vi "Load Process.vi"(0 "Object name":string, 3 "timeout (ms)":i32=10000, 5 "error in (no error)":errorcluster) -> (19 "error out":errorcluster)   [LabVIEW 2014, in "PTUtils.lvlib"]
uses:
  PTUtils.lvlib
  CS_Core/CSSystem/CoreDefs/CoreDefs.call_type.ctl
  CS_Core/BaseProcess/BaseProcess.descriptor string definition.ctl
  CS_Core/CSSystem/CoreDefs/CoreDefs.rawDataType.ctl
  CS_Core/CSSystem/CoreLib/CoreLib.string 2 byte array.vi
  CS_Core/CSSystem/CoreLib/CoreLib.lvlib
  CS_Core/CSSystem/CSSystemLib/CSSystemLib.lvlib
  CS_Core/BaseProcess/BaseProcess.lvlib
panel:
  in  "call cluster":T1
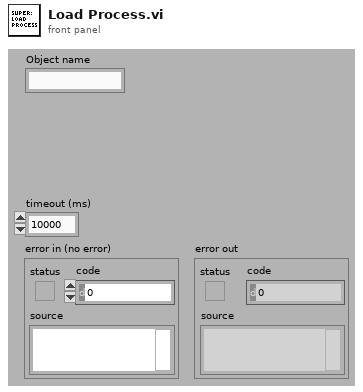
[diagram p1: front panel]
types:
  T1 = typedef "CoreDefs.call_type.ctl" = cluster{"Object":string, "Selector":string, "CallType":enum16{"simple", "synchronous", "asynchronous"}, "Async Object":string, "Async Selector":string, "Data Descriptor":T2, "Data":T3, "Error #":i32, "Expire":u32}
  T2 = typedef "BaseProcess.lvlib/BaseProcess.descriptor string definition.ctl" = string
  T3 = typedef "CoreDefs.rawDataType.ctl" = i8[]
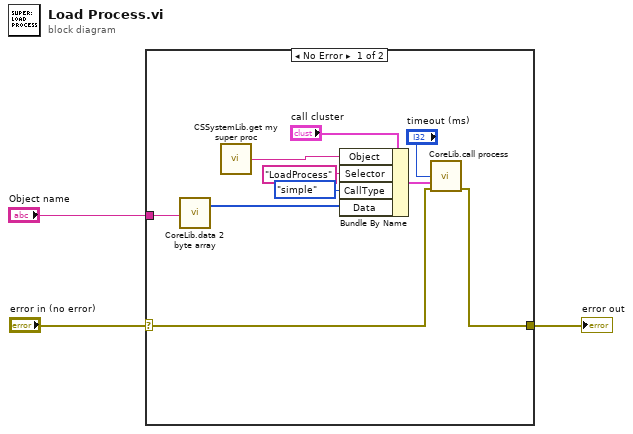
[diagram p0: block diagram]
diagram:
  n1 = case shown="No Error" "error in (no error)" {
    selector: "error in (no error)" -> [w6 w14]
    tunnel: "Object name" -> [w4 _]
    tunnel: [w5 w14] -> w1
    frame No Error {
      n2 = call-poly "CoreLib.data 2 byte array.vi"("string"=w4) -> ("byteArray out"=w13:T3)  [unwired: 18 in]
      n3 = call "CSSystemLib.get my super proc.vi"() -> ("name"=w10:string)  [unwired: 1 in]
      n4 = Bundle By Name(cluster="call cluster", "Object"=w10, "Selector"="LoadProcess", "CallType"=enum16{"simple", "synchronous", "asynchronous"}."simple", "Data"=w13) -> (w9:T1)
      n5 = call "CoreLib.call process.vi"("timeout (ms)"="timeout (ms)", "call cluster in"=w9, "error in (no error)"=w6) -> ("error out"=w5:errorcluster)  [unwired: 11 in, 1 out]
    }
    frame Error {
    }
  }
  "error out" <- w1
